vi "__allan[NORMALIZATION].vi"(3 "入力配列":dbl[][](array[numeric]), 5 "数値":i32=10) -> (0 "アラン分散/平均：　この値がアラン分散":dbl, 1 "アラン分散":dbl, 2 "時間間隔":dbl)   [LabVIEW 2017]
uses:
  <vilib>/Analysis/NI_AALBase.lvlib
panel:
  out "出力配列":dbl[][](array[numeric])
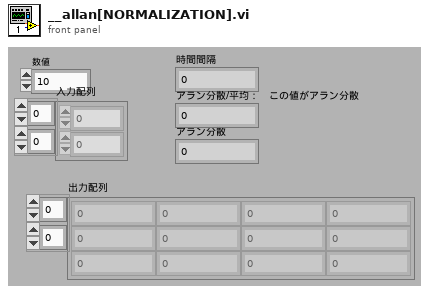
[diagram p1: front panel]
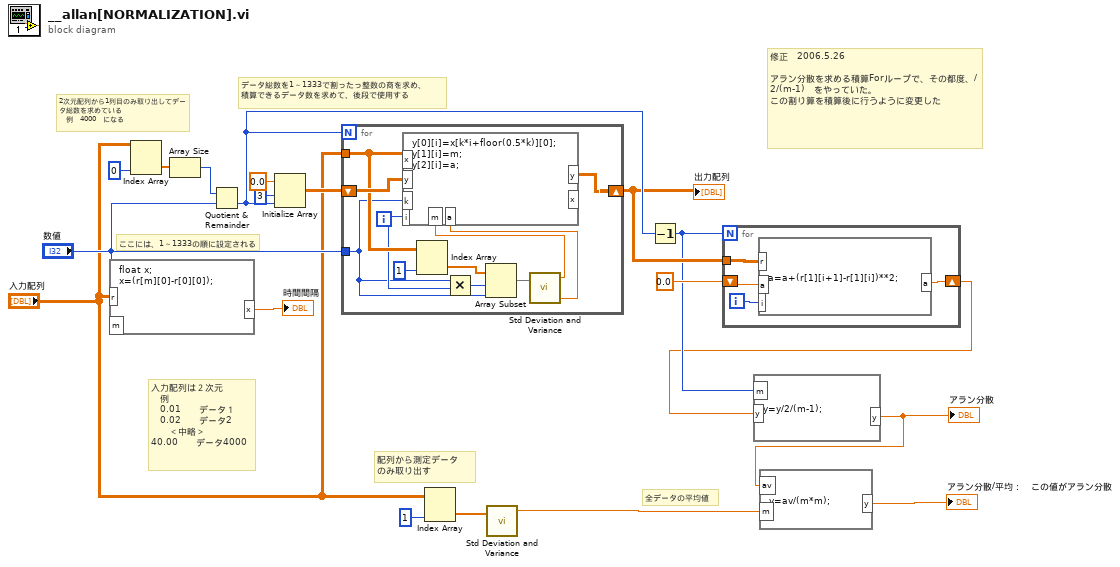
[diagram p0: block diagram]
diagram:
  # "データ総数を1～1333で割ったっ整数の商を求め、\n積算できるデータ数を求めて、後段で使用する"
  # "2次元配列から1列目のみ取り出してデータ総数を求めている\n　例　4000　になる"
  # "ここには、1～1333の順に設定される"
  # "入力配列は２次元\n　例\n　0.01　　データ１\n　0.02　　データ2\n　　＜中略＞\n40.00　　データ4000"
  # "配列から測定データ\nのみ取り出す"
  # "全データの平均値"
  # "修正　2006.5.26\n\nアラン分散を求める積算Forループで、その都度、/2/(m-1)　をやっていた。\nこの割り算を積算後に行うように変更した"
  n1 = formula code="float x;\nx=(r[m][0]-r[0][0]);"("r"="入力配列", "m"="数値") -> ("x"=→"時間間隔":dbl)
  n2 = Index Array(array="入力配列", index (col)=0) -> (element=w8:dbl[])  [unwired: 1 in]
  n3 = Array Size(array=w8) -> (size(s)=w16:i32)
  n4 = Quotient & Remainder(x=w16, y="数値") -> (floor(x/y)=w15:i32)  [unwired: 1 out]
  n5 = Initialize Array(0.0, 3, w15) -> (w18:dbl[][])
  n6 = for {
    N: w15 -> [_]
    tunnel: "数値" -> [w24]
    tunnel: "入力配列" -> [w28]
    shift-right: [w21] -> w13
    shift-left: w18 -> [w30]
    i -> [w25]
    n7 = Index Array(array=w28, index (col)=1) -> (element=w27:dbl[])  [unwired: 1 in]
    n8 = Multiply(x=w24, y=w25) -> (x*y=w23:i32)
    n9 = Array Subset(array=w27, index=w23, length=w24) -> (w29:dbl[])
    n10 = call <vilib>:"Std Deviation and Variance.vi"("X"=w29) -> ("mean"=w26:dbl, "variance"=w22:dbl)  [unwired: 1 in, 1 out]
    n11 = formula code="y[0][i]=x[k*i+floor(0.5*k)][0];\ny[1][i]=m;\ny[2][i]=a;"("x"=w28, "y"=w30, "i"=w25, "k"=w24, "m"=w26, "a"=w22) -> ("y"=w21:dbl[][])  [unwired: 1 out]
  }
  "出力配列" <- w13
  n12 = Index Array(array="入力配列", index (col)=1) -> (element=w5:dbl[])  [unwired: 1 in]
  n13 = call <vilib>:"Std Deviation and Variance.vi"("X"=w5) -> ("mean"=w10:dbl)  [unwired: 1 in, 2 out]
  n14 = Decrement(x=w15) -> (x-1=w3:i32)
  n15 = for {
    N: w3 -> [_]
    tunnel: w13 -> [w34]
    shift-right: [w31] -> w2
    shift-left: 0.0 -> [w33]
    i -> [w32]
    n16 = formula code="a=a+(r[1][i+1]-r[1][i])**2;"("r"=w34, "a"=w33, "i"=w32) -> ("a"=w31:dbl)
  }
  n17 = formula code="y=y/2/(m-1);"("m"=w3, "y"=w2) -> ("y"=w1:dbl)
  "アラン分散" <- w1
  n18 = formula code="y=av/(m*m);"("av"=w1, "m"=w10) -> ("y"=→"アラン分散/平均：　この値がアラン分散":dbl)
